vi "Get Firmware Builds Base Path.vi"(8 "Error In":errorcluster) -> (0 "Error Out":errorcluster, 3 "Firmware Builds Base Path":path)   [LabVIEW 2020, in "LMH-LINX.lvlib"]
doc: "Read Firmware Builds Base Path From .ini"
uses:
  LMH-LINX.lvlib
  <vilib>/Utility/config.llb/Read Key (Path).vi
  <vilib>/Utility/config.llb/NI_LVConfig.lvlib
  Toolbox/LMH-Toolbox.lvlib
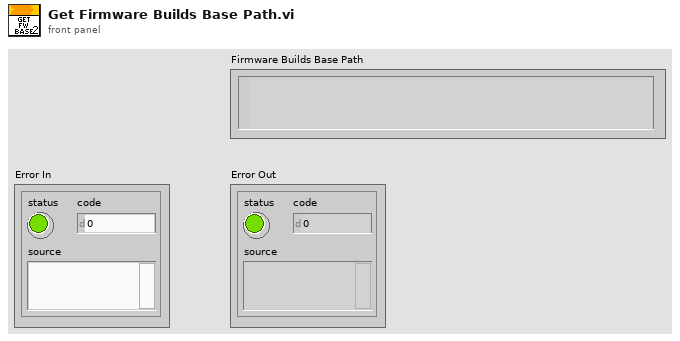
[diagram p1: front panel]
types:
  T1 = typedef "NI_LVConfig.lvlib/Config Data RefNum.ctl" = refnum<k1>
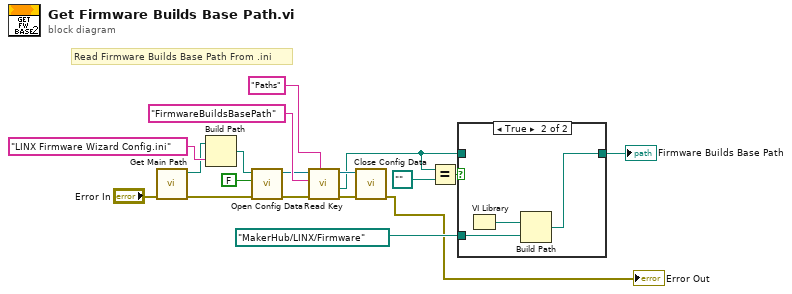
[diagram p0: block diagram]
diagram:
  # "Read Firmware Builds Base Path From .ini"
  n1 = call "Get Main Path.vi"("Error In"="Error In") -> ("Error Out"=w7:errorcluster, "Main Dir"=w10:path)  [unwired: 8 in, 1 out]
  n2 = Build Path(base path=w10, name or relative path="LINX Firmware Wizard Config.ini") -> (appended path=w9:path)
  n3 = call <vilib>:"Open Config Data.vi"("error in (no error)"=w7, "create file if necessary (T)"=FALSE, "configuration file path"=w9) -> ("error out"=w14:errorcluster, "refnum"=w15:T1)  [unwired: 6 in, 1 out]
  n4 = call-poly <vilib>:"Read Key.vi"("section"="Paths", "error in (no error)"=w14, "key"="FirmwareBuildsBasePath", "refnum"=w15) -> ("error out"=w13:errorcluster, "value"=w3:path, "refnum out"=w12:T1)  [unwired: 4 in, 1 out]
  n5 = call <vilib>:"Close Config Data.vi"("error in (no error)"=w13, "refnum"=w12) -> ("error out"=→"Error Out":errorcluster)  [unwired: 8 in, 1 out]
  n6 = Equal?(x=w3, y=path "" ("value")) -> (x = y?=w4:bool)
  n7 = case shown="True" w4 {
    tunnel: path "MakerHub/LINX/Firmware" -> [_ w22]
    tunnel: [w19 w20] -> w5
    tunnel: w3 -> [w19 _]
    frame False {
    }
    frame True {
      n8 = VI Library() -> (path=w21:path)
      n9 = Build Path(base path=w21, name or relative path=w22) -> (appended path=w20:path)
    }
  }
  "Firmware Builds Base Path" <- w5
